vi "acq.saveAcqParams.vi"(5 "camera in":refnum<class "camera.lvclass">, 7 "File name":string, 8 "error in":errorcluster, 10 "# Acq":u16, 11 "path":path) -> (0 "error out":errorcluster)   [LabVIEW 2020]
uses:
  camera/camera.lvclass
  <vilib>/Utility/file.llb/Write Delimited Spreadsheet (string).vi
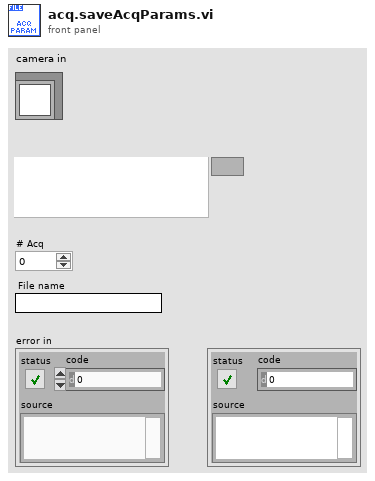
[diagram p1: front panel]
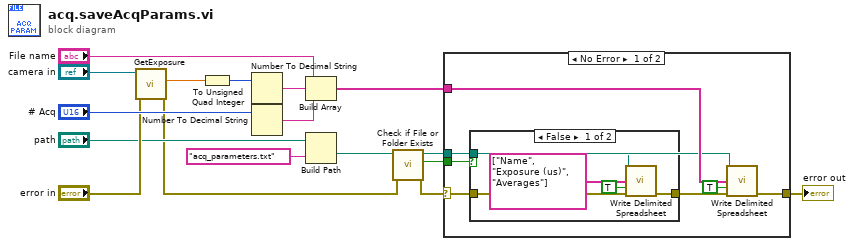
[diagram p0: block diagram]
diagram:
  n1 = call "GetExposure.vi"("error in"="error in", "camera.nit_c in"="camera in") -> ("error out"=w5:errorcluster, "exposure"=w16:dbl)  [unwired: 8 in]
  n2 = To Unsigned Quad Integer(1:w16) -> (0:w1:u64)
  n3 = Number To Decimal String(number=w1) -> (decimal integer string=w17:string)  [unwired: 1 in]
  n4 = Number To Decimal String(number="# Acq") -> (decimal integer string=w8:string)  [unwired: 1 in]
  n5 = Build Array("File name", w17, w8) -> (w10:string[])
  n6 = Build Path(base path="path", name or relative path="acq_parameters.txt" ("format string")) -> (appended path=w6:path)
  n7 = call <vilib>:"Check if File or Folder Exists.vi"("error in (no error)"=w5, "path"=w6) -> ("error out"=w3:errorcluster, "file or folder exists?"=w2:bool, "dup path"=w4:path)  [unwired: 7 in]
  n8 = case shown="No Error" w3 {
    selector: w3 -> [w20 w31]
    tunnel: w10 -> [w24 _]
    tunnel: [w23 w31] -> w9
    tunnel: w4 -> [w18 _]
    tunnel: w2 -> [w21 _]
    frame No Error {
      n9 = case shown="False" w21 {
        tunnel: w20 -> [w27 w30]
        tunnel: [w28 w30] -> w19
        tunnel: w18 -> [w26 _]
        frame False {
          n10 = call-poly <vilib>:"Write Delimited Spreadsheet.vi"("file path (dialog if empty)"=w26, "1D data"=string[] ["Name", "Exposure (us)", "Averages"] ("format string"), "append to file? (new file:F)"=TRUE, "error in (no error)"=w27) -> ("error out"=w28:errorcluster)  [unwired: 10 in, 1 out]
        }
        frame True {
        }
      }
      n11 = call-poly <vilib>:"Write Delimited Spreadsheet.vi"("file path (dialog if empty)"=w18, "1D data"=w24, "append to file? (new file:F)"=TRUE, "error in (no error)"=w19) -> ("error out"=w23:errorcluster)  [unwired: 10 in, 1 out]
    }
    frame Error {
    }
  }
  "error out" <- w9
